vi "testLoopbackUDP.vi"(8 "error in (no error)":errorcluster, 11 "TestCase in":refnum<class "DSF CD UDP System Tests.lvclass">) -> (0 "error out":errorcluster, 3 "TestCase out":refnum<class "DSF CD UDP System Tests.lvclass">)   [LabVIEW 2017, in "DSF CD UDP System Tests.lvclass"]
uses:
  DSF CD UDP System Tests.lvclass
  C:/Git/niveristand-custom-device-testing-tools/VeriStandTestCase/VeriStandTestCase.lvclass
  b55b5565-dc34-4e51-bcfa-5a6cba25043e.vi
  df0c3853-f0b6-44a9-ad36-32614d313efc.vi
  <vilib>/NI Veristand/Execution/Workspace/NI VeriStand - Set Single Channel Value.vi
  <vilib>/NI Veristand/Execution/Workspace/NI VeriStand - Get Single Channel Value.vi
  <vilib>/addons/_JKI Toolkits/VI Tester/TestCase.llb/TestCase.lvclass
  <vilib>/NI VeriStand/Execution/Workspace/NI_VS Workspace ExecutionAPI.lvlib
  C:/Program Files (x86)/National Instruments/LabVIEW 2017/vi.lib/addons/_JKI Toolkits/VI Tester/TestCase.llb/TestCase.lvclass
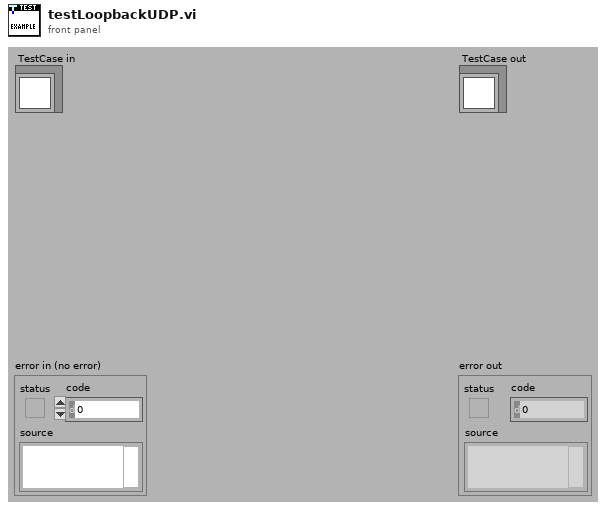
[diagram p1: front panel]
types:
  T1 = typedef "NI_VS Workspace ExecutionAPI.lvlib/WorkspaceAPI.ctl" = refnum<k24>
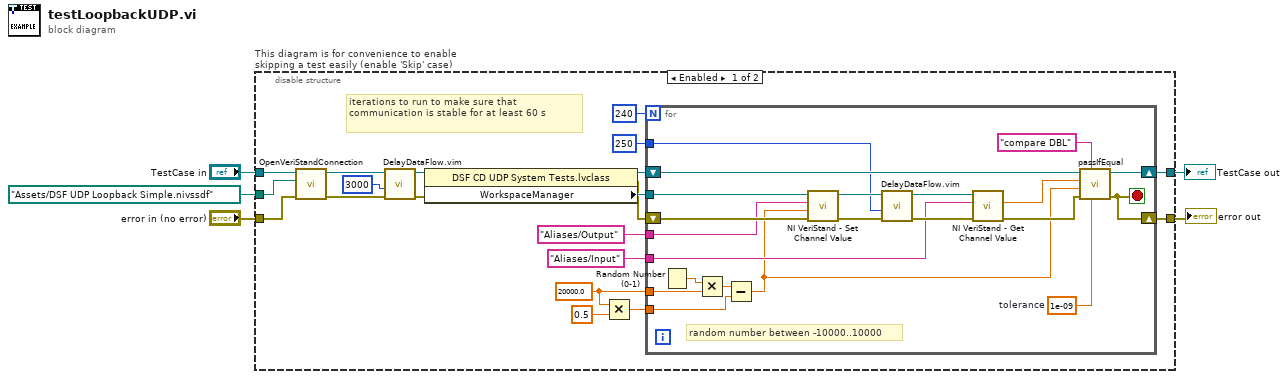
[diagram p0: block diagram]
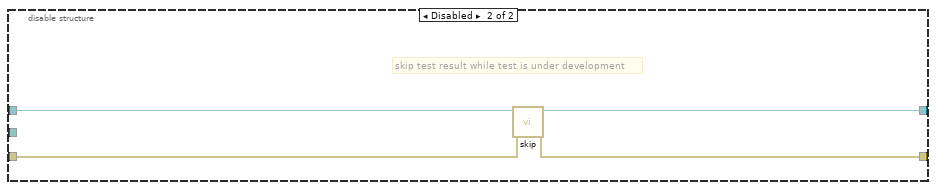
[diagram p2: hidden frame]
diagram:
  n1 = disable-structure "This diagram is for convenience to enable skipping a test easily (enable 'Skip' case)" shown="Enabled" {
    disable-tunnel: "TestCase in" -> [w23 w48]
    disable-tunnel: [w16 w46] -> w2
    disable-tunnel: [w15 w47] -> w4
    disable-tunnel: "error in (no error)" -> [w24 w45]
    disable-tunnel: path "Assets/DSF UDP Loopback Simple.nivssdf" ("System Definition File") -> [w11 _]
    frame Enabled {
      w7 = 20000.0 ("y")
      # "iterations to run to make sure that communication is stable for at least 60 s"
      n2 = call-dynamic "OpenVeriStandConnection.vi"("error in (no error)"=w24, "System Definition File"=w11, "VeriStand Test Case in"=w23) -> ("error out"=w13:errorcluster, "VeriStand Test Case out"=w22:refnum<class "DSF CD UDP System Tests.lvclass">)  [unwired: 6 in, 1 out]
      n3 = call "DelayDataFlow.vim"("value in"=w13, "milliseconds to wait"=u32 3000) -> ("value out"=w12:errorcluster)  [unwired: 2 in, 1 out]
      n4 = property class="DSF CD UDP System Tests.lvclass"(reference=w22, error in=w12) -> (reference out=w17:refnum<class "DSF CD UDP System Tests.lvclass">, error out=w20:errorcluster, "WorkspaceManager"=w21:T1)
      n5 = Multiply(x=w7, y=0.5) -> (x*y=w8:dbl)
      n6 = for {
        N: 240 -> [_]
        tunnel: w21 -> [w44]
        tunnel: "Aliases/Input" ("Channel") -> [w39]
        tunnel: "Aliases/Output" ("Channel") -> [w38]
        shift-right: [w25] -> w15
        shift-left: w20 -> [w43]
        shift-right: [w34] -> w16
        shift-left: w17 -> [w35]
        tunnel: w8 -> [w28]
        tunnel: w7 -> [w27]
        tunnel: u32 250 ("milliseconds to wait") -> [w26]
        stop <- w25 stop-if-true
        w30 = 1e-09  # tolerance
        # "random number between -10000..10000"
        n7 = Random Number (0-1)() -> (number: 0 to 1=w33:dbl)
        n8 = Multiply(x=w33, y=w27) -> (x*y=w32:dbl)
        n9 = Subtract(x=w32, y=w28) -> (x-y=w31:dbl)
        n10 = call-poly <vilib>:"NI VeriStand - Set Channel Value.vi"("error in (no error)"=w43, "Value"=w31, "Channel"=w38, "WorkspaceManager in"=w44) -> ("error out"=w42:errorcluster, "WorkspaceManager out"=w40:T1)  [unwired: 6 in]
        n11 = call "DelayDataFlow.vim"("value in"=w42, "milliseconds to wait"=w26) -> ("value out"=w41:errorcluster)  [unwired: 2 in, 1 out]
        n12 = call-poly <vilib>:"NI VeriStand - Get Channel Value.vi"("error in (no error)"=w41, "Channel"=w39, "WorkspaceManager in"=w40) -> ("error out"=w37:errorcluster, "Value"=w36:dbl)  [unwired: 6 in, 1 out]
        n13 = call-dynamic "passIfEqual.vi"("delta (optional)"=w30, "custom report message (\"\")"="compare DBL" ("custom report message (\"\")"), "error in (no error)"=w37, "y"=w31, "x"=w36, "TestCase in"=w35) -> ("error out"=w25:errorcluster, "TestCase out"=w34:refnum<class "DSF CD UDP System Tests.lvclass">)  [unwired: 4 in]
      }
    }
    frame Disabled {
      # "skip test result while test is under development"
      n14 = call <vilib>:"skip.vi"("error in (no error)"=w45, "TestCase in"=w48) -> ("error out"=w47:errorcluster, "TestCase out"=w46:refnum<class "DSF CD UDP System Tests.lvclass">)  [unwired: 8 in]
    }
  }
  "error out" <- w4
  "TestCase out" <- w2
